vi "HMIDataHTTPGet.vi"(7 "LabVIEW Web Service Request":refnum<class "Web Request.lvclass">) -> (2 "JSON string":string)   [LabVIEW 2019]
uses:
  <vilib>/wsapi/Web Request.lvclass
panel:
  # "Use the Web Service Request input terminal to call the VIs on the Web Services palette. Do not remove it from the connector pane unless you don't need access to the palette."
  # "Each additional control wired to the connector pane will be available as an input in the URL. To include an indicator in terminal-mode output (the default setting), it must also be wired to the connector pane."
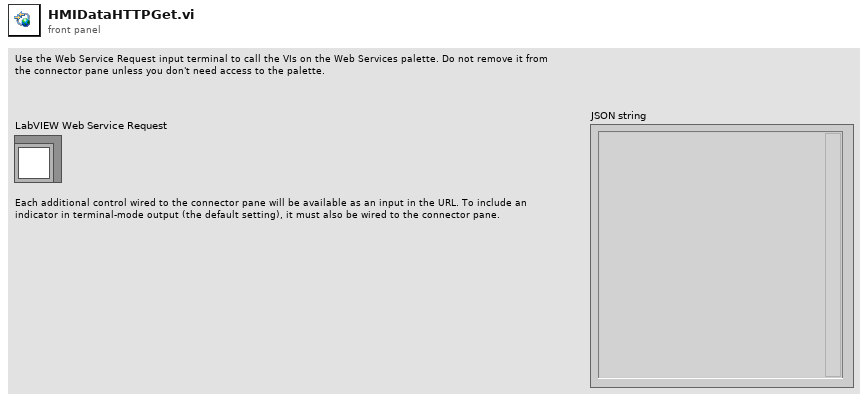
[diagram p1: front panel]
types:
  T1 = typedef "HMI Typedef.ctl" = cluster{"Current Latitude":dbl, "Current Longitude":dbl, "Separation Distance":dbl, "Global Stop":bool, "UTC Offset Valid":bool, "1 Hz INS Out":dbl[], "GNSS Fix Status":u32, "satellites available":u8, "System Status Array":string[], "Enable Sys Clock Update":bool, "Spatial Dual Timestamp (External)":u64, "SD Filter Status":bool[], "SD System Status":bool[], "FPGA Time Acquired":bool}
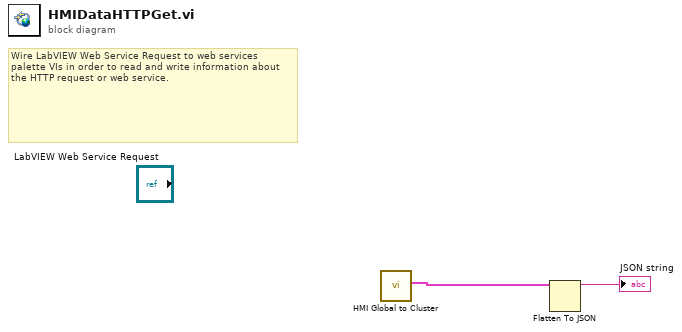
[diagram p0: block diagram]
diagram:
  # "Wire LabVIEW Web Service Request to web services palette VIs in order to read and write information about the HTTP request or web service."
  n1 = call "HMI Global to Cluster.vi"() -> ("HMI Cluster Out"=w1:T1)  [unwired: 10 in]
  n2 = Flatten To JSON(anything=w1) -> (JSON string=→"JSON string":string)  [unwired: 2 in, 1 out]
